vi "OFDM_modulator_proj.vi"(4 "error in (no error)":errorcluster, 5 "OFDM Parameters":T1={"FFT size (N)"=64, "Length of CP (Lc)"=8, "Null Tones"=[0, 30, 31, 32], "Training Sequence FFT size"=1, "Training Sequence Length of CP"=0, "Number of OFDM symbols (derived)"=0}, 7 "input symbols":cdb[](array[numeric])) -> (0 "error out":errorcluster, 1 "OFDM Parameters out":T1={"FFT size (N)"=64, "Length of CP (Lc)"=8, "Null Tones"=[0, 30, 31, 32], "Training Sequence FFT size"=1, "Training Sequence Length of CP"=0, "Number of OFDM symbols (derived)"=0}, 3 "output samples":cdb[](array[numeric]))   [LabVIEW 2013]
uses:
  OFDM_parameters.ctl
  <vilib>/Analysis/2dsp.llb/Inverse Complex FFT.vi
  <vilib>/Analysis/NI_AALPro.lvlib
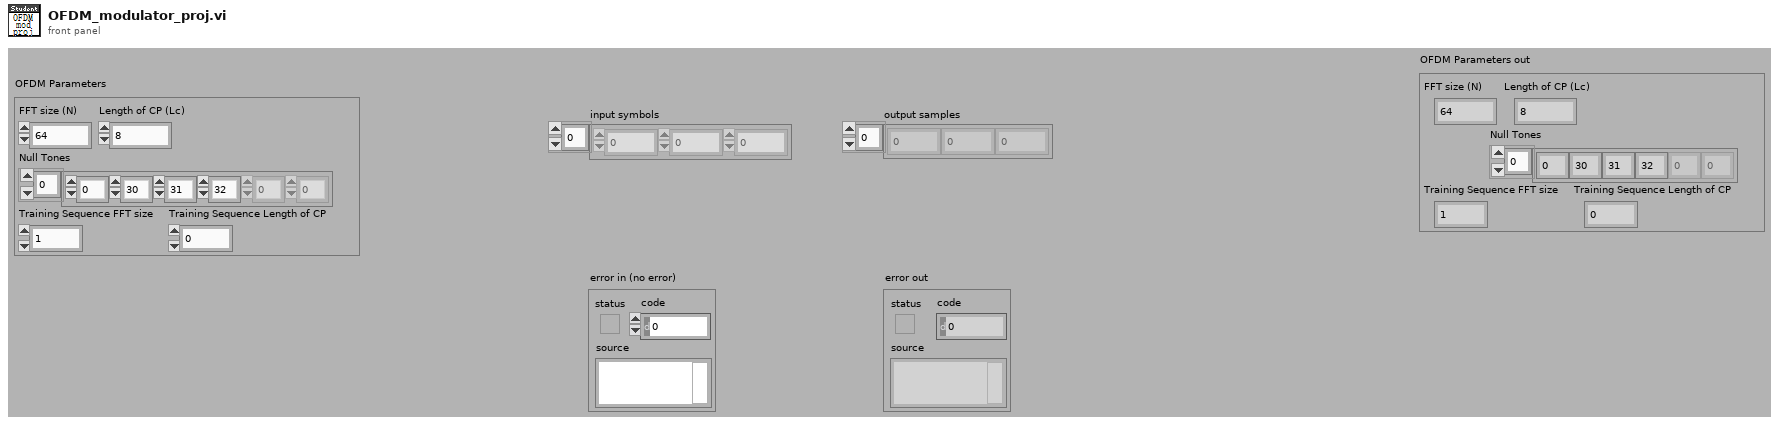
[diagram p1: front panel]
types:
  T1 = typedef "OFDM_parameters.ctl" = cluster{"FFT size (N)":i32, "Length of CP (Lc)":i32, "Null Tones":u32[], "Training Sequence FFT size":i32, "Training Sequence Length of CP":i32, "Number of OFDM symbols (derived)":i32}
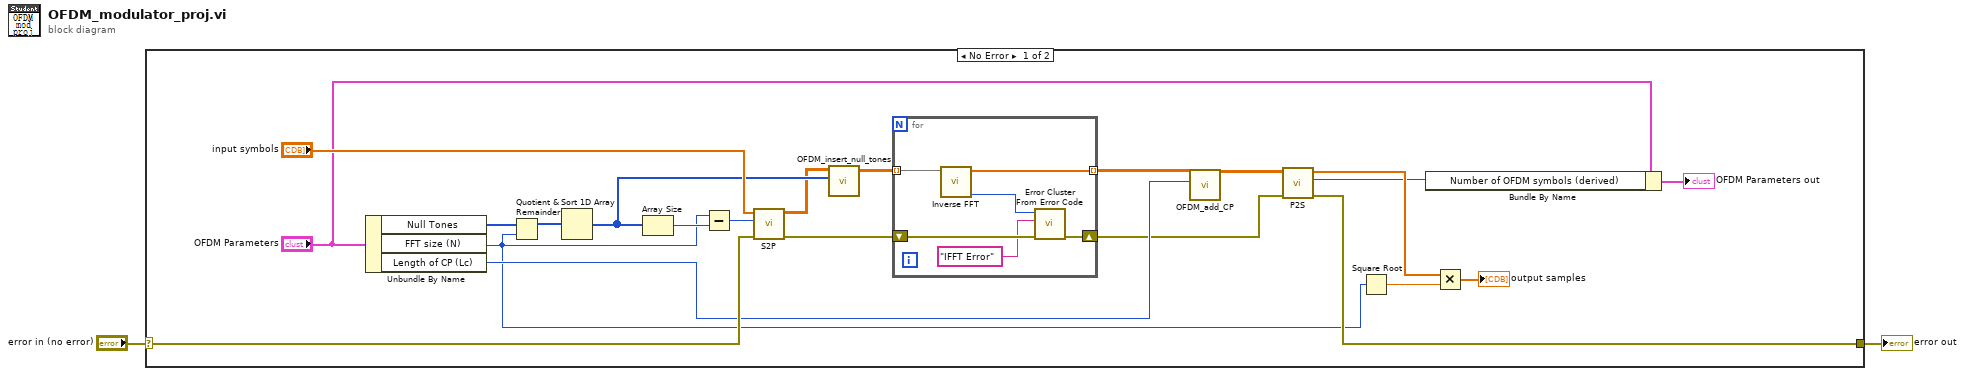
[diagram p0: block diagram]
diagram:
  n1 = case shown="No Error" "error in (no error)" {
    selector: "error in (no error)" -> [w15 w31]
    tunnel: [w10 w31] -> w1
    frame No Error {
      n2 = Unbundle By Name("OFDM Parameters") -> ("Null Tones"=w24:u32[], "FFT size (N)"=w3:i32, "Length of CP (Lc)"=w13:i32)
      n3 = Quotient & Remainder(x=w24, y=w3) -> (x-y*floor(x/y)=w23:u32[])  [unwired: 1 out]
      n4 = Sort 1D Array(array=w23) -> (sorted array=w19:u32[])
      n5 = Array Size(array=w19) -> (size(s)=w22:i32)
      n6 = Subtract(x=w3, y=w22) -> (x-y=w21:i32)
      n7 = call "S2P.vi"("error in (no error)"=w15, "block size"=w21, "serial input"="input symbols") -> ("error out"=w14:errorcluster, "parallel output"=w18:cdb[][])  [unwired: 3 in]
      n8 = call "OFDM_insert_null_tones.vi"("null tones"=w19, "input"=w18) -> ("output"=w17:cdb[][])  [unwired: 5 in]
      n9 = for {
        tunnel: w17 -> [w30] mode=indexing
        tunnel: [w29] -> w16 mode=indexing
        shift-right: [w28] -> w11
        shift-left: w14 -> [w27]
        n10 = call-poly <vilib>:"Inverse FFT.vi"("FFT {X}"=w30) -> ("error"=w26:i32, "X"=w29:cdb[])  [unwired: 9 in]
        n11 = call <vilib>:"Error Cluster From Error Code.vi"("error in (no error)"=w27, "error message (\"\")"="IFFT Error", "error code (0)"=w26) -> ("error out"=w28:errorcluster)  [unwired: 6 in]
      }
      n12 = call "OFDM_add_CP.vi"("length of CP (Lc)"=w13, "input"=w16) -> ("output"=w12:cdb[][])  [unwired: 5 in]
      n13 = call "P2S.vi"("error in (no error)"=w11, "parallel input"=w12) -> ("error out"=w10:errorcluster, "block size"=w6:i32, "serial output"=w8:cdb[])  [unwired: 3 in]
      n14 = Square Root(x=w3) -> (sqrt(x)=w9:dbl)
      n15 = Bundle By Name(cluster="OFDM Parameters", "Number of OFDM symbols (derived)"=w6) -> (→"OFDM Parameters out":T1)
      n16 = Multiply(x=w8, y=w9) -> (x*y=→"output samples":cdb[])
    }
    frame Error {
    }
  }
  "error out" <- w1
